vi "Write Session manager service gRPC ID.vi"(8 "error in (no error)":errorcluster, 10 "gRPCid":T1, 11 "MeasurementContext in":refnum<class "MeasurementContext.lvclass">) -> (0 "error out":errorcluster, 3 "MeasurementContext out":refnum<class "MeasurementContext.lvclass">)   [LabVIEW 2020, in "MeasurementLink Measurement Server.lvlib" / "MeasurementContext.lvclass"]
uses:
  MeasurementContext.lvclass
  MeasurementContext.lvclass/MeasurementContext.ctl
  <vilib>/gRPC/LabVIEW gRPC Library/Shared/grpcId.ctl
  <vilib>/gRPC/LabVIEW gRPC Library/grpc-lvsupport-release.lvlib
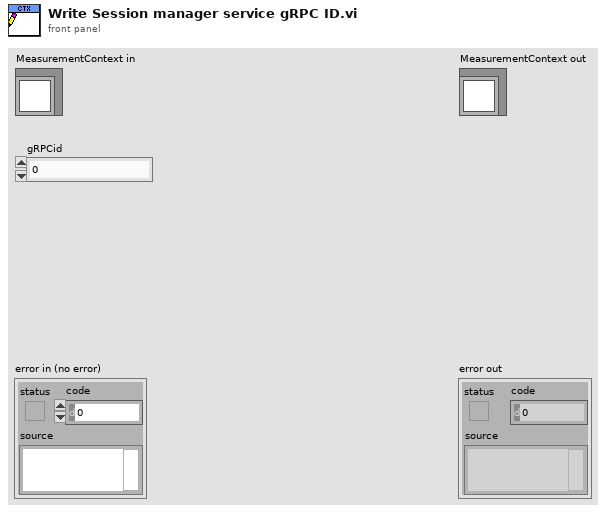
[diagram p1: front panel]
types:
  T1 = typedef "grpc-lvsupport-release.lvlib/grpcId.ctl" = u64
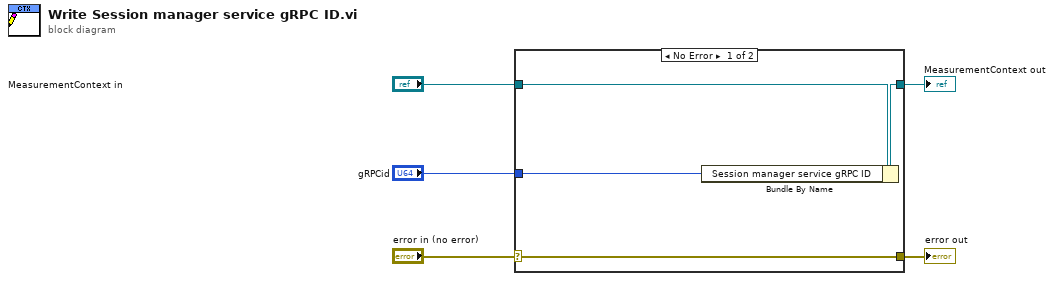
[diagram p0: block diagram]
diagram:
  n1 = case shown="No Error" "error in (no error)" {
    selector: "error in (no error)" -> [w9 w10]
    tunnel: [w9 w10] -> w4
    tunnel: [w7 w11] -> w2
    tunnel: "MeasurementContext in" -> [w8 w11]
    tunnel: "gRPCid" -> [w6 _]
    frame No Error {
      n2 = Bundle By Name(cluster=w8, "Session manager service gRPC ID"=w6) -> (w7:refnum<class "MeasurementContext.lvclass">)
    }
    frame Error {
    }
  }
  "error out" <- w4
  "MeasurementContext out" <- w2
